vi "Export_Get Device List.vi"(11 "Export Setting":T1[](array[typedef])) -> (3 "Device Names":string[](array[string]))   [LabVIEW 2015, in "ConfigHelper.lvlib"]
uses:
  ConfigHelper.lvlib
  Control_Export Setup.ctl
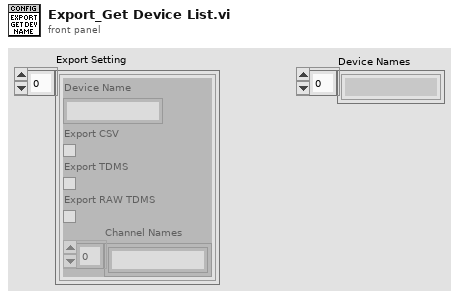
[diagram p1: front panel]
types:
  T1 = typedef "ConfigHelper.lvlib/Control_Export Setup.ctl" = cluster{"Device Name":string, "Export CSV":bool, "Export TDMS":bool, "Export RAW TDMS":bool, "Channel Names":string[]}
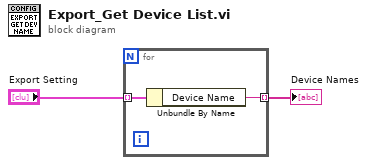
[diagram p0: block diagram]
diagram:
  n1 = for {
    tunnel: "Export Setting" -> [w4] mode=indexing
    tunnel: [w3] -> w1 mode=indexing
    n2 = Unbundle By Name(w4) -> ("Device Name"=w3:string)
  }
  "Device Names" <- w1
